vi "[RT] Finite Acq.vi"() -> ()   [LabVIEW 2015]
doc: "The finite acquisition mode tells the FPGA to acquire a certain number of samples and then terminate the acquisition. In this acquisition mode, the rwfm_ConfigTiming VI calls rwfm_BufferConfig.vi and sets the host application's data buffer size equal to the number of points in the finite acquisition."
uses:
  <vilib>/rvi/interface/nirviCloseFPGA/nirviCloseFPGA.xnode
  <vilib>/NI/cRIO Wfm/cRIO Wfm.lvlib
  <vilib>/NI/cRIO Wfm/AcqRead(Wfm).vi
  <vilib>/rvi/interface/nirviOpenFPGA/nirviOpenFPGA.xnode
  <vilib>/FPGAPlugInAG/cRIO-9074/niLvFpga_Open_cRIO-9074.vi
  <vilib>/rvi/interface/common/dynamic/niFpgaDynamicAddResources.vi
  <vilib>/FPGAPlugInAG/Dynamic/niLvFpga_Close_Dynamic.vi
  C:/Program Files (x86)/National Instruments/LabVIEW 2015/ProjectTemplates/Source/cRIOWfm/FPGA Bitfiles/DeltaSigMain_9074.lvbitx
  C:/Program Files (x86)/National Instruments/LabVIEW 2015/ProjectTemplates/Source/cRIOWfm/FPGA/[FPGA] DeltaSig Main.vi
  C:/Program Files (x86)/National Instruments/LabVIEW 2015/ProjectTemplates/Source/cRIOWfm/FPGA Bitfiles/SARAcqMain_9074.lvbitx
  C:/Program Files (x86)/National Instruments/LabVIEW 2015/ProjectTemplates/Source/cRIOWfm/FPGA/[FPGA] SAR Acq Main.vi
  <vilib>/NI/cRIO Wfm/ChannelConfig.ctl
panel:
  in  "Sample Rate":u32=51200
  in  "Channel Info":T1=[{"Channel Name"="Mod1/ai0", "Sensitivity mV_EU"=1000.0, "EU"="V", "dB Ref EU"=1.0}, {"Channel Name"="Mod1/ai1", "Sensitivity mV_EU"=1000.0, "EU"="V", "dB Ref EU"=1.0}, {"Channel Name"="Mod1/ai2", "Sensitivity mV_EU"=1000.0, "EU"="V", "dB Ref EU"=1.0}, {"Channel Name"="Mod1/ai3", "Sensitivity mV_EU"=1000.0, "EU"="V", "dB Ref EU"=1.0}] caption="Channel Name      Scale [mV/EU]        EU           dB Ref [EU]" {"dB Ref EU" format="%#.2p"; "Sensitivity mV_EU" format="%.2f"}
  out "Waveform Graph":waveform(sgl)[](graph)
  in  "Samps per Chan":i32=25600 caption="Samples per Channel"
  # "Sampling Info"
  # "Channel Info"
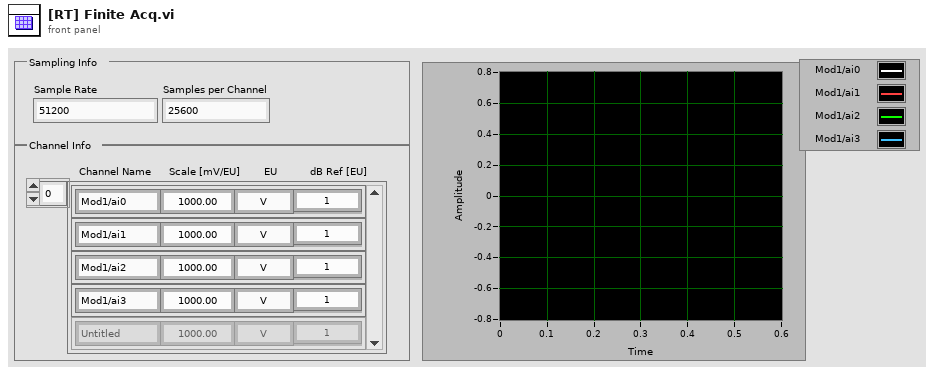
[diagram p1: front panel]
types:
  T1 = typedef "cRIO Wfm.lvlib/ChannelConfig.ctl" = cluster{"Channel Name":string, "Sensitivity mV_EU":dbl, "EU":string, "dB Ref EU":dbl}[]
  T2 = typedef "cRIO Wfm.lvlib/SamplingInfo.ctl" = cluster{"Number of Channels":i32, "Actual Samp Rate":dbl, "Chan Name Array":string[], "EU Chan Array":string[], "dB Ref Chan Array":dbl[]}
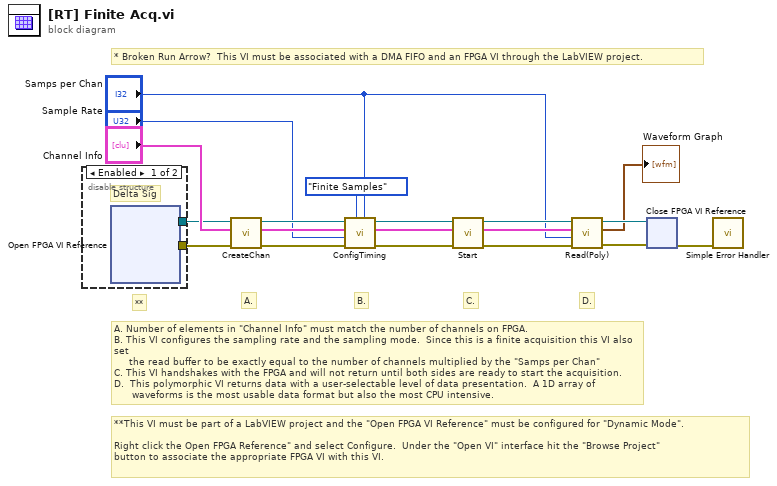
[diagram p0: block diagram]
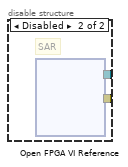
[diagram p2: hidden frame]
diagram:
  # "**This VI must be part of a LabVIEW project and the \"Open FPGA VI Reference\" must be configured for \"Dynamic Mode\".\n\nRight click the Open FPGA Reference\" and select Configure.  Under the \"Open VI\" interface hit the \"Browse Project\" \nbutton to associate the appropriate FPGA VI with this VI."
  # "* Broken Run Arrow?  This VI must be associated with a DMA FIFO and an FPGA VI through the LabVIEW project."
  # "A. Number of elements in \"Channel Info\" must match the number of channels on FPGA.\nB. This VI configures the sampling rate and the sampling mode.  Since this is a finite acquisition this VI also set  \n     the read buffer to be exactly equal to the number of channels multiplied by the \"Samps per Chan\"\nC. This VI handshakes with the FPGA and will not return until both sides are ready to start the acquisition.\nD.  This polymorphic VI returns data with a user-selectable level of data presentation.  A 1D array of     \n      waveforms is the most usable data format but also the most CPU intensive."
  # "**"
  # "D."
  # "C."
  # "B."
  # "A."
  n1 = disable-structure shown="Enabled" {
    disable-tunnel: [w21 w23] -> w2
    disable-tunnel: [w20 w22] -> w1
    frame Enabled {
      # "Delta Sig"
      n2 = xnode "Open FPGA VI Reference"() -> ("FPGA VI Reference Out"=w21:refnum<k20>, "error out"=w20:errorcluster)  [unwired: 2 in]
    }
    frame Disabled {
      # "SAR"
      n3 = xnode "Open FPGA VI Reference"() -> ("FPGA VI Reference Out"=w23:refnum<k20>, "error out"=w22:errorcluster)  [unwired: 2 in]
    }
  }
  n4 = call <vilib>:"CreateChan.vi"("error in"=w1, "Channel Info"="Channel Info", "Dynamic FPGA Ref"=w2) -> ("error out"=w16:errorcluster, "Sampling Info"=w15:T2, "Dynamic FPGA Ref Out"=w17:refnum<k20>)  [unwired: 1 in, 5 out]
  n5 = call <vilib>:"ConfigTiming.vi"("Samples per Channel"="Samps per Chan", "Sample Mode"=enum16{"Finite Samples", "Continuous Samples"}."Finite Samples", "error in"=w16, "Sample Rate"="Sample Rate", "Sampling Info In"=w15, "Dynamic FPGA Ref"=w17) -> ("error out"=w9:errorcluster, "Sampling Info Out"=w10:T2, "Dynamic FPGA Ref Out"=w11:refnum<k20>)  [unwired: 2 in, 1 out]
  n6 = call <vilib>:"Start.vi"("error in"=w9, "Sampling Info In"=w10, "Dynamic FPGA Ref"=w11) -> ("error out"=w13:errorcluster, "Sampling Info Out"=w14:T2, "Dynamic FPGA Ref Out"=w12:refnum<k20>)  [unwired: 6 out]
  n7 = call-poly <vilib>:"Read(Poly).vi"("error in"=w13, "Samps Read per Chan"="Samps per Chan", "Sampling Info"=w14, "Dynamic FPGA Ref"=w12) -> ("error out"=w7:errorcluster, "Wfm Data"=→"Waveform Graph":waveform(sgl)[], "Dynamic FPGA Ref Out"=w8:refnum<k20>)  [unwired: 2 in, 3 out]
  n8 = xnode "Close FPGA VI Reference"("FPGA VI Reference In"=w8, "error in"=w7) -> ("error out"=w18:errorcluster)
  n9 = call <vilib>:"Simple Error Handler.vi"("error in (no error)"=w18) -> ()  [unwired: 1 in, 8 out]
